vi "WPI_CounterOpen Gear Tooth Sensor Mode.vi"(4 "External Reset Active High":bool=TRUE, 6 "External Reset":T1={"DevStatus"={"status"=FALSE, "code"=0, "source"=""}, "AnalogTriggerMode?"=FALSE, "DigitalMode"={"DIO Channel"=enum."Disabled"}, "AnalogTriggerMode"={"AnalogTriggerIndex"=enum."Trig 0", "OutputType"=enum."InWindow"}}, 8 "error in (no error)":errorcluster, 9 "Invert Direction":bool, 10 "Direction Sensitive":bool, 11 "Source":T1={"DevStatus"={"status"=FALSE, "code"=0, "source"=""}, "AnalogTriggerMode?"=FALSE, "DigitalMode"={"DIO Channel"=enum."Disabled"}, "AnalogTriggerMode"={"AnalogTriggerIndex"=enum."Trig 0", "OutputType"=enum."InWindow"}}) -> (0 "error out":errorcluster, 3 "CounterDevRef":T5)   [LabVIEW 2017]
doc: "Opens a reference to a counter and configures the counter to detect pulses when a gear tooth passes the sensor.\n\nThis software is licensed. Open the labview\\readme\\WPI Robotics Library Open Source License.txt file for more information."
uses:
  <vilib>/Rock Robotics/SystemInterfaces/Counter/FPGA_CounterCtrEdgeDetectionType.ctl
  <vilib>/Rock Robotics/SystemInterfaces/Counter/FPGA_CounterCtrSystemIndex.ctl
  <vilib>/Rock Robotics/WPI/Counter/WPI_CounterDevRef.ctl
  <vilib>/Rock Robotics/SystemInterfaces/AnalogTrigger/FPGA_AnalogTriggerOutType.ctl
  <vilib>/Rock Robotics/SystemInterfaces/CounterEncoderSourceConvertion/FPGA_CounterEncoderSourceConvertionLVSourceType.ctl
  <vilib>/Rock Robotics/SystemInterfaces/DIO/FPGA_DIODigitalSourceChannel.ctl
  <vilib>/Rock Robotics/SystemInterfaces/AnalogTrigger/FPGA_AnalogTriggerIndex.ctl
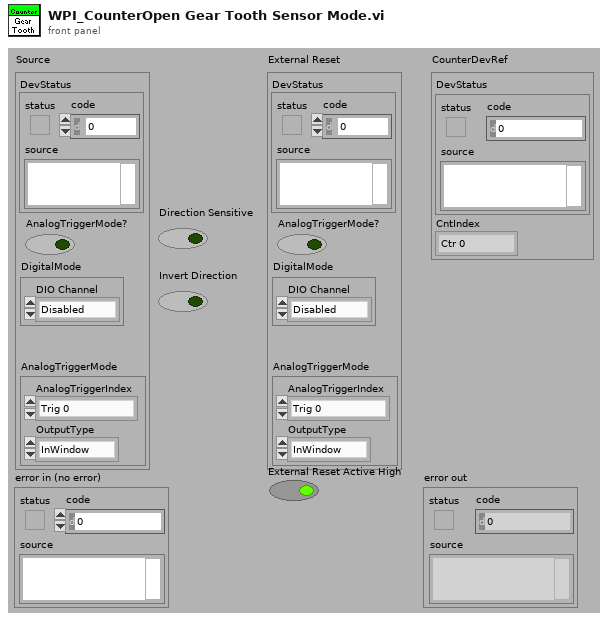
[diagram p1: front panel]
types:
  T1 = typedef "FPGA_CounterEncoderSourceConvertionLVSourceType.ctl" = cluster{"DevStatus":errorcluster, "AnalogTriggerMode?":bool, "DigitalMode":cluster{"DIO Channel":T2}, "AnalogTriggerMode":cluster{"AnalogTriggerIndex":T3, "OutputType":T4}}
  T2 = typedef "FPGA_DIODigitalSourceChannel.ctl" = enum8{"DIO 0", "DIO 1", "DIO 2", "DIO 3", "DIO 4", "DIO 5", "DIO 6", "DIO 7", "DIO 8", "DIO 9", "DIO MXP 0", "DIO MXP 1", "DIO MXP 2", "DIO MXP 3", "DIO MXP 4", "DIO MXP 5", "DIO MXP 6", "DIO MXP 7", "DIO MXP 8", "DIO MXP 9", "DIO MXP 10", "DIO MXP 11", "DIO MXP 12", "DIO MXP 13", "DIO MXP 14", "DIO MXP 15", "Disabled"}
  T3 = typedef "FPGA_AnalogTriggerIndex.ctl" = enum8{"Trig 0", "Trig 1", "Trig 2", "Trig 3", "Trig 4", "Trig 5", "Trig 6", "Trig 7", "Invalid"}
  T4 = typedef "FPGA_AnalogTriggerOutType.ctl" = enum16{"InWindow", "TriggerState", "Rising", "Falling"}
  T5 = typedef "WPI_CounterDevRef.ctl" = cluster{"DevStatus":errorcluster, "CntIndex":T6}
  T6 = typedef "FPGA_CounterCtrSystemIndex.ctl" = enum8{"Ctr 0", "Ctr 1", "Ctr 2", "Ctr 3", "Ctr 4", "Ctr 5", "Ctr 6", "Ctr 7", "Invalid"}
  T7 = typedef "FPGA_CounterCtrEdgeDetectionType.ctl" = cluster{"Master Mode":enum16{"Edge Detection", "Semi Period Mode", "Pulse Length Mode", "External Direction"}, "UpChannel":enum16{"Rising Edge", "Falling Edge", "Raising & Falling Edge", "Disabled"}, "DownChannel":enum16{"Rising Edge", "Falling Edge", "Raising & Falling Edge", "Disabled"}, "High/Up":bool}
  T8 = enum16{"Edge Detection", "Semi Period Mode", "Pulse Length Mode", "External Direction"}
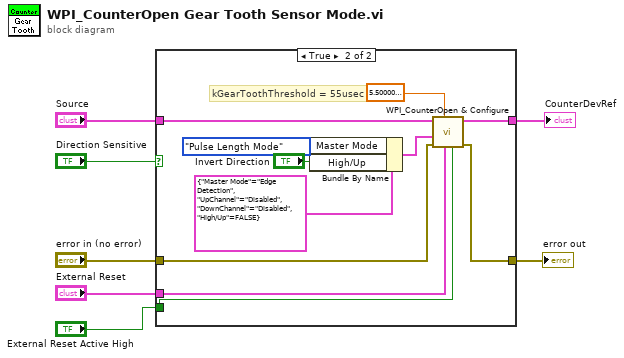
[diagram p0: block diagram]
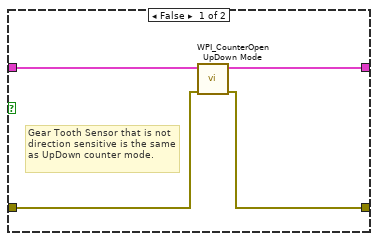
[diagram p2: hidden frame]
diagram:
  n1 = case shown="True" "Direction Sensitive" {
    tunnel: "Source" -> [w8 w21]
    tunnel: "error in (no error)" -> [w9 w19]
    tunnel: [w10 w18] -> w5
    tunnel: [w11 w17] -> w4
    tunnel: "External Reset" -> [_ w13]
    tunnel: "External Reset Active High" -> [_ w12]
    frame False {
      # "Gear Tooth Sensor that is not direction sensitive is the same as UpDown counter mode."
      n2 = call <vilib>:"WPI_CounterOpen UpDown Mode.vi"("error in (no error)"=w9, "Up Source"=w8) -> ("error out"=w10:errorcluster, "CounterDevRef"=w11:T5)  [unwired: 5 in, 3 out]
    }
    frame True {
      # "kGearToothThreshold = 55usec"
      n3 = Bundle By Name(cluster=T7 {"Master Mode"=enum."Edge Detection", "UpChannel"=enum."Disabled", "DownChannel"=enum."Disabled", "High/Up"=FALSE} ("EdgeType"), "Master Mode"=T8."Pulse Length Mode", "High/Up"="Invert Direction") -> (w20:T7)
      n4 = call <vilib>:"WPI_CounterOpen & Configure.vi"("External Reset Trigger"=w12, "External Reset"=w13, "GTSDirThreshold"=sgl 5.5e-05, "error in (no error)"=w19, "EdgeType"=w20, "Up Source"=w21) -> ("error out"=w18:errorcluster, "CounterDevRef"=w17:T5)  [unwired: 1 in, 3 out]
    }
  }
  "CounterDevRef" <- w4
  "error out" <- w5
